vi "Get UID.vi"(8 "error in (no error)":errorcluster, 11 "Object Layout in":refnum<class "Object Layout.lvclass">) -> (0 "error out":errorcluster, 2 "UID":i32, 3 "Object Layout out":refnum<class "Object Layout.lvclass">)   [LabVIEW 2010, in "NI_SE_Front Panel Layout.lvlib" / "Object Layout.lvclass"]
uses:
  Object Layout.lvclass
  Object Layout.lvclass/Object Layout.ctl
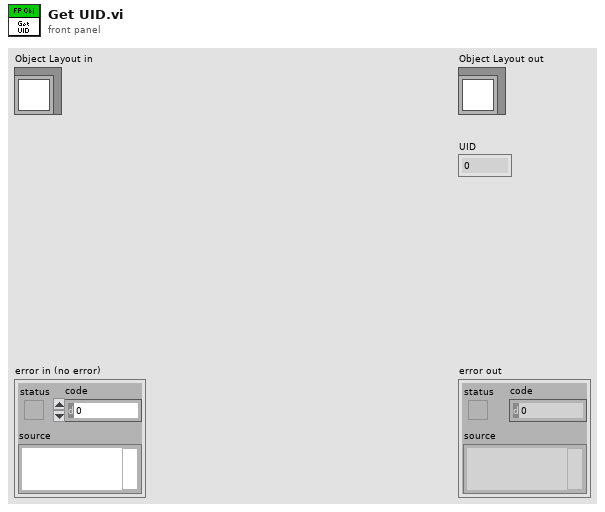
[diagram p1: front panel]
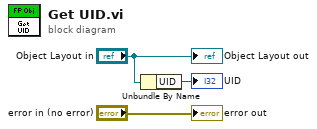
[diagram p0: block diagram]
diagram:
  n1 = Unbundle By Name("Object Layout in") -> ("UID"=→"UID":i32)
  "error out" <- "error in (no error)"
  "Object Layout out" <- "Object Layout in"
